vi "Log Error.vi"(8 "error in (no error)":errorcluster, 11 "Application Controller in":refnum<class "Application Controller.lvclass">) -> (0 "error out":errorcluster, 1 "Error message":string, 2 "stop actor?":bool=TRUE, 3 "Application Controller out":refnum<class "Application Controller.lvclass">, 4 "LabActor Error":T1)   [LabVIEW 2020, in "Application Controller.lvclass"]
uses:
  Application Controller.lvclass
  C:/GitHub/LabActor/Template Module/Template Module.lvclass
  Template Module/LabActor Error.ctl
  <vilib>/Utility/sysdir.llb/System Directory Type.ctl
  <vilib>/Utility/error.llb/DialogType.ctl
  Template Module/Template Module.lvclass/Template Module.ctl
  Template Module/Read Name.vi
  Template Module/Read Report error and stop.vi
  <vilib>/Utility/error.llb/Error Cluster From Error Code.vi
  <vilib>/ErrorRing/Error Ring.xnode
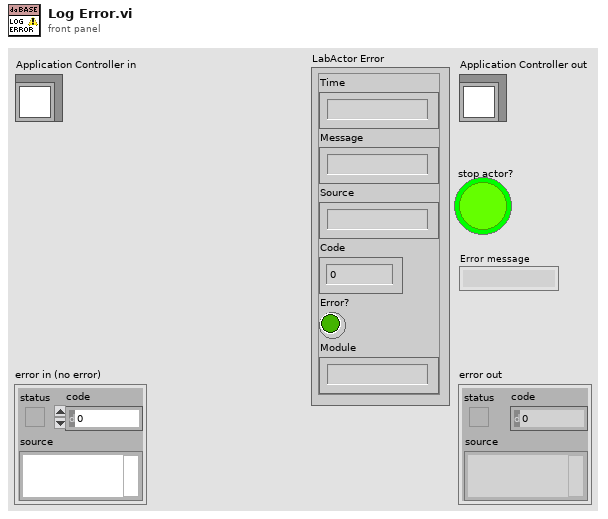
[diagram p1: front panel]
types:
  T1 = typedef "LabActor Error.ctl" = cluster{"Time":string, "Message":string, "Source":string, "Code":i32, "Error?":bool, "Module":string}
  T2 = enum16{"open", "replace", "create", "open or create", "replace or create", "replace or create with confirmation"}
  T3 = typedef "DialogType.ctl" = u16
  T4 = typedef "System Directory Type.ctl" = i32
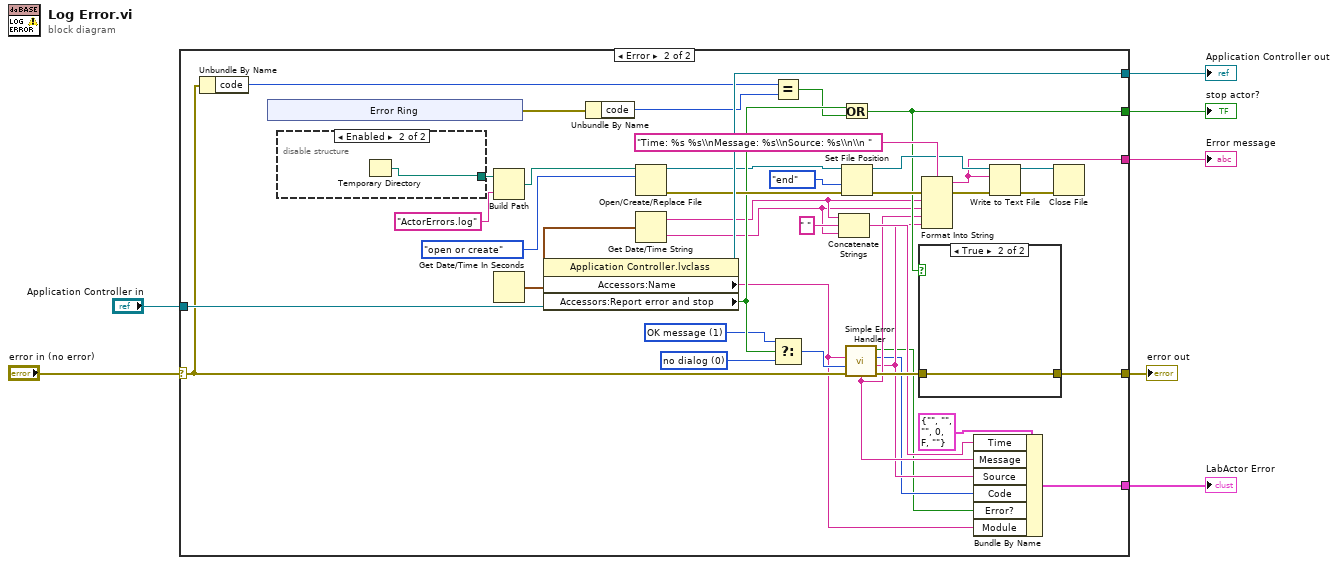
[diagram p0: block diagram]
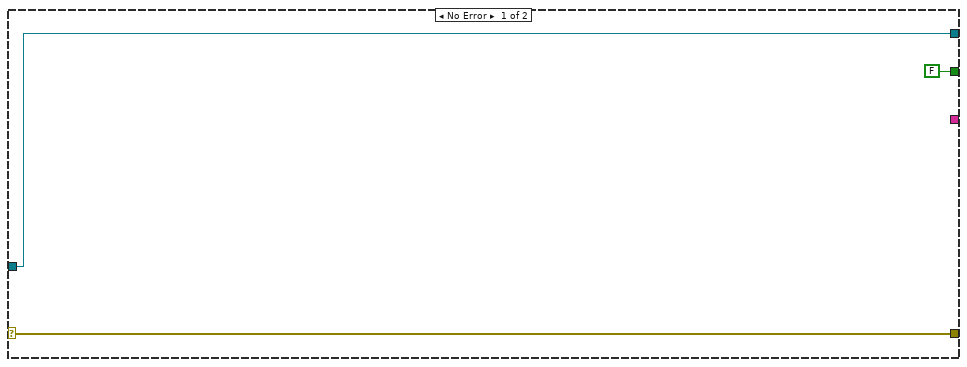
[diagram p2: hidden frame]
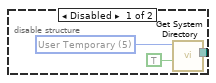
[diagram p3: hidden frame]
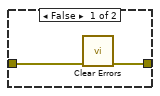
[diagram p4: hidden frame]
diagram:
  n1 = case shown="Error" "error in (no error)" {
    selector: "error in (no error)" -> [w9 w47]
    tunnel: [w9 w33] -> w6
    tunnel: [w10 w49] -> w4
    tunnel: "Application Controller in" -> [w10 w50]
    tunnel: [FALSE ("Accessors:Report error and stop") w23] -> w3
    tunnel: [_ w27] -> w2
    tunnel: [_ w16] -> w1
    frame No Error {
    }
    frame Error {
      w25 = T3 1 items=["no dialog", "OK message", "continue or stop message", "OK message + warnings", "continue/stop + warnings"] ("type of dialog (OK msg:1)")
      w26 = T3 0 items=["no dialog", "OK message", "continue or stop message", "OK message + warnings", "continue/stop + warnings"] ("type of dialog (OK msg:1)")
      n2 = Unbundle By Name(w47) -> ("code"=w46:i32)
      n3 = xnode "Error Ring"() -> ("error out"=w48:errorcluster)
      n4 = disable-structure shown="Enabled" {
        disable-tunnel: [w51 w54] -> w44
        frame Disabled {
          w53 = T4 5 items=["User Home"=0, "User Desktop"=1, "User Documents"=2, "User Application Data"=3, "User Preferences"=4, "User Temporary"=5, "Public Documents"=6, "Public Application Data"=7, "Public Preferences"=8, "Public Cache"=13, "System Core Libraries"=9, "System Installed Libraries"=10, "Application Files"=11, "Boot Volume Root"=12] ("system directory type")
          n5 = call <vilib>:"Get System Directory.vi"("create directory if not found? (F)"=TRUE, "system directory type"=w53) -> ("system directory"=w51:path)  [unwired: 9 in]
        }
        frame Enabled {
          n6 = Temporary Directory() -> (w54:path)
        }
      }
      n7 = Build Path(base path=w44, name or relative path="ActorErrors.log") -> (appended path=w42:path)
      n8 = Get Date/Time In Seconds() -> (seconds since 1Jan1904=w39:timestamp)
      n9 = property class="Application Controller.lvclass"(reference=w50) -> (reference out=w49:refnum<class "Application Controller.lvclass">, "Accessors:Name"=w11:string, "Accessors:Report error and stop"=w32:bool)  [unwired: 1 in, 1 out]
      n10 = Unbundle By Name(w48) -> ("code"=w45:i32)
      n11 = Open/Create/Replace File(file path (use dialog)=w42, operation (0:open)=T2."open or create") -> (refnum out=w30:refnum<file>, error out=w38:errorcluster)  [unwired: 4 in, 1 out]
      n12 = Get Date/Time String(seconds (now)=w39) -> (date string=w19:string, time string=w17:string)  [unwired: 2 in]
      n13 = Equal?(x=w46, y=w45) -> (x = y?=w22:bool)
      n14 = Select(t=w25, s=w32, f=w26) -> (s? t:f=w24:T3)
      n15 = Concatenate Strings(w19, " " ("string"), w17) -> (w20:string)
      n16 = Or(x=w32, y=w22) -> (x .or. y?=w23:bool)
      n17 = Set File Position(refnum=w30, from (0:start)=enum16{"start", "end", "current"}."end", error in=w38) -> (refnum out=w29:refnum<file>, error out=w31:errorcluster)  [unwired: 1 in]
      n18 = call <vilib>:"Simple Error Handler.vi"("error source (\" \")"=w11, "type of dialog (OK msg:1)"=w24, "error in (no error)"=w47) -> ("error?"=w12:bool, "code out"=w13:i32, "source out"=w14:string, "error out"=w34:errorcluster, "message"=w15:string)  [unwired: 2 in]
      n19 = case shown="True" w23 {
        tunnel: w34 -> [w56 w57]
        tunnel: [w55 w57] -> w33
        frame False {
          n20 = call <vilib>:"Clear Errors.vi"("error in (no error)"=w56) -> ("error out"=w55:errorcluster)  [unwired: 5 in, 1 out]
        }
        frame True {
        }
      }
      n21 = Format Into String(format string="Time: %s %s\\nMessage: %s\\nSource: %s\\n\\n ", error in=w31, w19, w17, w15, w14) -> (resulting string=w27:string, error out=w37:errorcluster)  [unwired: 1 in]
      n22 = Bundle By Name(cluster=T1 {"Time"="", "Message"="", "Source"="", "Code"=0, "Error?"=FALSE, "Module"=""} ("LabActor Error"), "Time"=w20, "Message"=w15, "Source"=w14, "Code"=w13, "Error?"=w12, "Module"=w11) -> (w16:T1)
      n23 = Write to Text File(file (use dialog)=w29, text=w27, error in=w37) -> (refnum out=w36:refnum<file>, error out=w35:errorcluster)  [unwired: 1 in, 1 out]
      n24 = Close File(refnum=w36, error in=w35) -> ()  [unwired: 2 out]
    }
  }
  "error out" <- w6
  "Application Controller out" <- w4
  "stop actor?" <- w3
  "Error message" <- w2
  "LabActor Error" <- w1
